vi "fit-cluster.vi"(1 "Image In":T2, 2 "donnees fit":T1) -> (0 "F - baseline  (pN)":dbl)   [LabVIEW 2019]
uses:
  <vilib>/vision/Image Controls.llb/IMAQ Image.ctl
  <vilib>/Analysis/NI_AALPro.lvlib
  <vilib>/vision/NI_Vision_Development_Module.lvlib
panel:
  # "SORTIES"
  # "ENTREES"
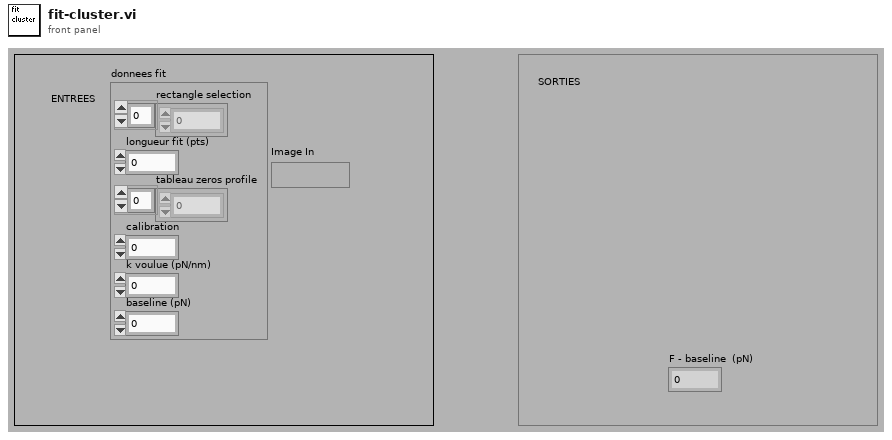
[diagram p1: front panel]
types:
  T1 = cluster{"rectangle selection":i32[], "longueur fit (pts)":i32, "tableau zeros profile":dbl[], "calibration":dbl, "k voulue (pN/nm)":dbl, "baseline (pN)":dbl}
  T2 = typedef "IMAQ Image.ctl" = refnum<image>
  T3 = enum32{"SVD", "Givens", "Givens2", "Householder", "LU Decomposition", "Cholesky"}
  T4 = cluster{"Polynomial Coefficients[0]":dbl, "Polynomial Coefficients[1]":dbl, "Polynomial Coefficients[2]":dbl, "Polynomial Coefficients[3]":dbl, "Polynomial Coefficients[4]":dbl, "Polynomial Coefficients[5]":dbl, "Polynomial Coefficients[6]":dbl, "Polynomial Coefficients[7]":dbl, "Polynomial Coefficients[8]":dbl}
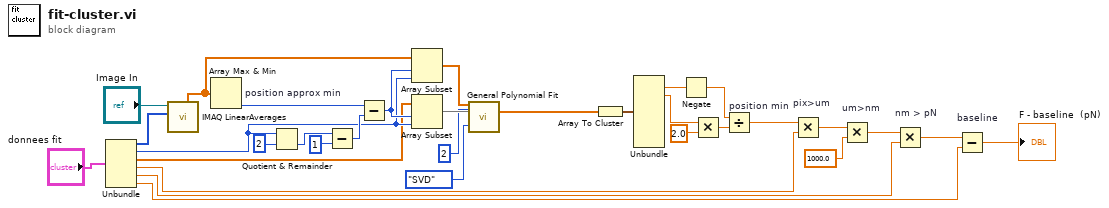
[diagram p0: block diagram]
diagram:
  n1 = Unbundle("donnees fit") -> ("rectangle selection"=w6:i32[], "longueur fit (pts)"=w5:i32, "tableau zeros profile"=w4:dbl[], "calibration"=w3:dbl, "k voulue (pN/nm)"=w2:dbl, "baseline (pN)"=w1:dbl)
  n2 = call "IMAQ LinearAverages"("Optional Rectangle"=w6, "Image Src"="Image In") -> ("X Axis Averages"=w16:sgl[])  [unwired: 2 in, 7 out]
  n3 = Array Max & Min "position approx min"(array=w16) -> (min index (indices)=w30:i32)  [unwired: 3 out]
  n4 = Quotient & Remainder(x=w5, y=2) -> (floor(x/y)=w32:i32)  [unwired: 1 out]
  n5 = Subtract(x=w32, y=1) -> (x-y=w29:i32)
  n6 = Subtract(x=w30, y=w29) -> (x-y=w28:i32)
  n7 = Array Subset(array=w16, index=w28, length=w5) -> (w15:sgl[])
  n8 = Array Subset(array=w4, index=w28, length=w5) -> (w26:dbl[])
  n9 = call <vilib>:"General Polynomial Fit.vi"("Y"=w15, "polynomial order"=2, "X"=w26, "algorithm"=T3."SVD") -> ("Polynomial Coefficients"=w23:dbl[])  [unwired: 8 in, 3 out]
  n10 = Array To Cluster(array=w23) -> (cluster=w22:T4)
  n11 = Unbundle(w22) -> ("Polynomial Coefficients[1]"=w21:dbl, "Polynomial Coefficients[2]"=w17:dbl)  [unwired: 7 out]
  n12 = Negate(x=w21) -> (-x=w20:dbl)
  n13 = Multiply(x=w17, y=2.0) -> (x*y=w19:dbl)
  n14 = Divide "position min"(x=w20, y=w19) -> (x/y=w11:dbl)
  n15 = Multiply "pix>um"(x=w11, y=w3) -> (x*y=w13:dbl)
  n16 = Multiply "um>nm"(x=w13, y=1000.0) -> (x*y=w14:dbl)
  n17 = Multiply "nm > pN"(x=w14, y=w2) -> (x*y=w10:dbl)
  n18 = Subtract "baseline"(x=w10, y=w1) -> (x-y=→"F - baseline  (pN)":dbl)
